vi "OFDM-SIM频偏校正.vi"(1 "采样频率":dbl, 2 "索引":i32, 3 "频偏":dbl[](array[numeric]), 4 "每个OFDM符号":cdb[](array[numeric])) -> (0 "校正频偏后OFDM符号":cdb[](array[numeric]))   [LabVIEW 2018]
uses:
  <vilib>/Analysis/1siggen.llb/Ramp Pattern by Samples.vi
  <vilib>/Analysis/NI_AALBase.lvlib
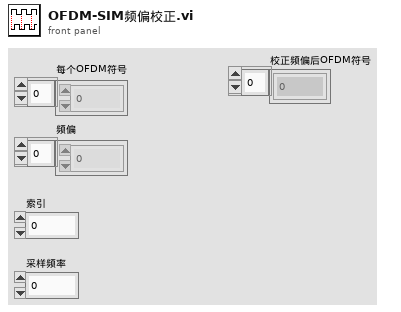
[diagram p1: front panel]
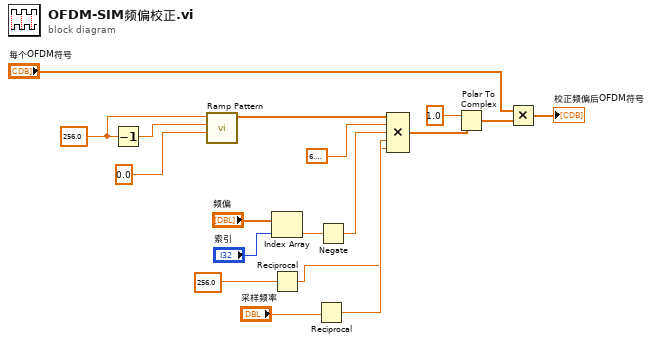
[diagram p0: block diagram]
diagram:
  w15 = 256.0 ("x")
  n1 = Decrement(x=w15) -> (x-1=w14:dbl)
  n2 = call-poly <vilib>:"Ramp Pattern.vi"("start"=0.0, "end"=w14, "samples"=w15) -> ("Ramp Pattern"=w12:dbl[])  [unwired: 7 in, 1 out]
  n3 = Index Array(array="频偏", index="索引") -> (element=w16:dbl)
  n4 = Reciprocal(x=256.0) -> (1/x=w1:dbl)
  n5 = Reciprocal(x="采样频率") -> (1/x=w3:dbl)
  n6 = Negate(x=w16) -> (-x=w9:dbl)
  n7 = Compound Arithmetic op=MULTIPLY(w12, 6.283185307179586, w9, w3, w1) -> (w10:dbl[])
  n8 = Polar To Complex(1:w10, 2:1.0) -> (0:w7:cdb[])
  n9 = Multiply(x="每个OFDM符号", y=w7) -> (x*y=→"校正频偏后OFDM符号":cdb[])
